vi "statistics.vi"() -> ()   [LabVIEW 2012]
uses:
  meas_date.vi
panel:
  out "Array":dbl[](array[numeric])
  out "odchyl":dbl
  out "œrednia":dbl
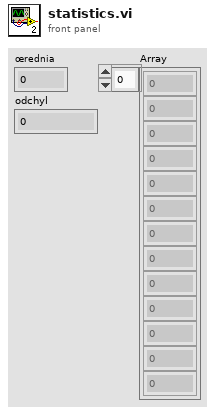
[diagram p1: front panel]
types:
  T1 = cluster{"No.":u64, "Voltage":dbl, "Current":dbl, "time":dbl, "Temperature":dbl}[]
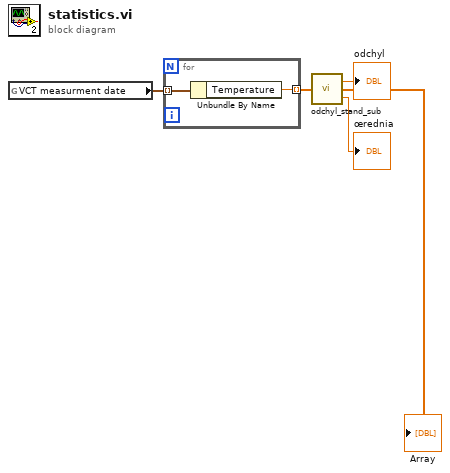
[diagram p0: block diagram]
diagram:
  n1 = global read "meas_date.vi" "VCT measurment date"() -> (w4:T1)
  n2 = for {
    tunnel: w4 -> [w6] mode=indexing
    tunnel: [w5] -> w3 mode=indexing
    n3 = Unbundle By Name(w6) -> ("Temperature"=w5:dbl)
  }
  "Array" <- w3
  n4 = call "odchyl_stand_sub.vi"("próbka"=w3) -> ("odchyl"=→"odchyl":dbl, "œrednia"=→"œrednia":dbl)
